vi "Test write read.vi"() -> ()   [LabVIEW 2021]
uses:
  TypeDefs/Read Configuration.ctl
  TypeDefs/Read Position.ctl
  TypeDefs/Data Element Details.ctl
  2e8eb7a4-6c45-41fc-8a56-8b93f8ab2aed.vi
  1e1cc0e0-5587-4368-b9c8-22ab8a2609bf.vi
  124ed0cf-21a2-4029-8b72-d8b2bc3cfca2.vi
  5f672ce3-c1c3-4239-be86-591df5452e6b.vi
  7cfac513-7288-4c82-908e-0b73a446185f.vi
  0aeae9fb-4646-413c-b569-2ea3bfc416eb.vi
  83090dc5-7c38-4dd0-9690-bbdffacb842e.vi
  30ab5228-805b-4106-80f0-7bddeadb9d94.vi
  0f7b4db4-c933-4198-9d44-a71b046c91fc.vi
  fd82cae6-90a1-4db4-8629-0dfa001c7628.vi
  3a8d97a0-d580-4512-a7c4-2f0697e6c9e2.vi
  132e0870-f3bc-4a70-93a8-8291f934a74e.vi
  1a26c85e-4bdf-40ac-9bb8-9f3aeb47762f.vi
  fc566840-9c7d-4747-891b-faea8883fc20.vi
  4087863d-db22-4010-a15b-9626b6b88f25.vi
  5d30ffee-c7bc-441f-904d-ba5baae4ab9b.vi
  5997d33c-b1c7-4e50-8cd9-5e7827217409.vi
  1b0a551c-ab50-4056-a338-be00ced168a1.vi
  1475facd-0be5-4a16-b5c0-d4b4098ff17d.vi
  2d2b7dd1-084a-416f-9403-29da1a0cacdf.vi
  71538749-b1ea-46d3-91f5-b8a08187b131.vi
  7ca0a5c6-c913-495e-bc60-1e54ff021bc4.vi
  0c9d9d69-203a-4c45-ab83-8723ccfac58a.vi
  8b09acb3-1804-4adb-b57a-6ab97de36fae.vi
  41820140-f02b-403e-8f6d-e5d8cc9e6038.vi
  5fe378b5-e28f-447f-911b-385a06e12749.vi
  6975467f-3c1c-408b-9985-6bf92f704002.vi
  a5ee0e2d-1d32-4a5c-9f8c-ab7e37a9bb32.vi
  6e041348-7f94-4adb-a506-9e6ae80f31c7.vi
  287dc7c8-fd1f-4848-acac-6b048d61fa92.vi
  96fd03da-6166-4d98-b503-d6d912d62be1.vi
  cd5f71e7-aa80-496b-a46f-ff9cfb96c09e.vi
  ab81dfaa-b4ed-4dad-90db-c2069a499ab9.vi
  cdd1d806-cf03-48b9-80a7-5abb69cc969c.vi
  934c8ee6-8108-47c3-ab0c-e7f3872857de.vi
  0617b4dd-75f0-4fc1-be0a-72d777f45d9a.vi
  6dbf1ba6-5076-4e89-aafa-fa0408d53c9c.vi
  87883e52-c370-4e1d-99dd-8208e79277b9.vi
  5a5884df-cfb3-4237-a45a-462ccf1dc42e.vi
  d4ea617a-d912-406f-a3a4-9dbd6f53576b.vi
  305478fb-600b-4089-8c06-0e062707fa97.vi
  44847041-c2b7-4435-a919-9d7ef56b5811.vi
  442734bb-6a94-4929-a174-6a0af52723c3.vi
  37e1ea89-1b34-4e4e-9bfd-fc0f3fde4930.vi
  2b752281-b4de-4725-8373-b94f73551aa8.vi
  2e8eb7a4-6c45-41fc-8a56-8b93f8ab2aed.vi/49b3dd2d-4579-4089-b72e-3f0875c862f2.vi
  SubVIs/Check Error.vi
  SubVIs/Get dll Path.vi
  SubVIs/Get Element Write Position.vi
  SubVIs/Notify Of New Write.vi
  124ed0cf-21a2-4029-8b72-d8b2bc3cfca2.vi/ad4ed45e-f2aa-403d-a38b-be52afbcecdf.vi
  5f672ce3-c1c3-4239-be86-591df5452e6b.vi/49b3dd2d-4579-4089-b72e-3f0875c862f2.vi
  0aeae9fb-4646-413c-b569-2ea3bfc416eb.vi/ad4ed45e-f2aa-403d-a38b-be52afbcecdf.vi
  83090dc5-7c38-4dd0-9690-bbdffacb842e.vi/bd07d5d9-1209-45ad-b636-9e9ab86132fb.vi
  0f7b4db4-c933-4198-9d44-a71b046c91fc.vi/ad4ed45e-f2aa-403d-a38b-be52afbcecdf.vi
  fd82cae6-90a1-4db4-8629-0dfa001c7628.vi/bd07d5d9-1209-45ad-b636-9e9ab86132fb.vi
  132e0870-f3bc-4a70-93a8-8291f934a74e.vi/ad4ed45e-f2aa-403d-a38b-be52afbcecdf.vi
  1a26c85e-4bdf-40ac-9bb8-9f3aeb47762f.vi/49b3dd2d-4579-4089-b72e-3f0875c862f2.vi
  4087863d-db22-4010-a15b-9626b6b88f25.vi/ad4ed45e-f2aa-403d-a38b-be52afbcecdf.vi
  5d30ffee-c7bc-441f-904d-ba5baae4ab9b.vi/ad4ed45e-f2aa-403d-a38b-be52afbcecdf.vi
  5997d33c-b1c7-4e50-8cd9-5e7827217409.vi/49b3dd2d-4579-4089-b72e-3f0875c862f2.vi
  2d2b7dd1-084a-416f-9403-29da1a0cacdf.vi/ad4ed45e-f2aa-403d-a38b-be52afbcecdf.vi
  71538749-b1ea-46d3-91f5-b8a08187b131.vi/ad4ed45e-f2aa-403d-a38b-be52afbcecdf.vi
  7ca0a5c6-c913-495e-bc60-1e54ff021bc4.vi/49b3dd2d-4579-4089-b72e-3f0875c862f2.vi
  41820140-f02b-403e-8f6d-e5d8cc9e6038.vi/ad4ed45e-f2aa-403d-a38b-be52afbcecdf.vi
  5fe378b5-e28f-447f-911b-385a06e12749.vi/ad4ed45e-f2aa-403d-a38b-be52afbcecdf.vi
  6975467f-3c1c-408b-9985-6bf92f704002.vi/49b3dd2d-4579-4089-b72e-3f0875c862f2.vi
  6e041348-7f94-4adb-a506-9e6ae80f31c7.vi/ad4ed45e-f2aa-403d-a38b-be52afbcecdf.vi
  287dc7c8-fd1f-4848-acac-6b048d61fa92.vi/ad4ed45e-f2aa-403d-a38b-be52afbcecdf.vi
  96fd03da-6166-4d98-b503-d6d912d62be1.vi/49b3dd2d-4579-4089-b72e-3f0875c862f2.vi
  ab81dfaa-b4ed-4dad-90db-c2069a499ab9.vi/ad4ed45e-f2aa-403d-a38b-be52afbcecdf.vi
  cdd1d806-cf03-48b9-80a7-5abb69cc969c.vi/49b3dd2d-4579-4089-b72e-3f0875c862f2.vi
  0617b4dd-75f0-4fc1-be0a-72d777f45d9a.vi/ad4ed45e-f2aa-403d-a38b-be52afbcecdf.vi
  6dbf1ba6-5076-4e89-aafa-fa0408d53c9c.vi/49b3dd2d-4579-4089-b72e-3f0875c862f2.vi
  87883e52-c370-4e1d-99dd-8208e79277b9.vi/49b3dd2d-4579-4089-b72e-3f0875c862f2.vi
  5a5884df-cfb3-4237-a45a-462ccf1dc42e.vi/49b3dd2d-4579-4089-b72e-3f0875c862f2.vi
  SubVIs/Wait For N Elements Available.vi
  SubVIs/Get Element Read Position.vi
  SubVIs/Set Element Read Position.vi
  442734bb-6a94-4929-a174-6a0af52723c3.vi/49b3dd2d-4579-4089-b72e-3f0875c862f2.vi
  2b752281-b4de-4725-8373-b94f73551aa8.vi/ad4ed45e-f2aa-403d-a38b-be52afbcecdf.vi
  <vilib>/Utility/error.llb/Trim Whitespace.vi
  <vilib>/string/Create NI GUID.vi
  <vilib>/Utility/error.llb/Error Cluster From Error Code.vi
  SubVIs/Get Element Info Variant.vi
  CIF_NI_CIPC.lvlib
panel:
  out "status":string
  out "pass":bool
  out "error out":errorcluster
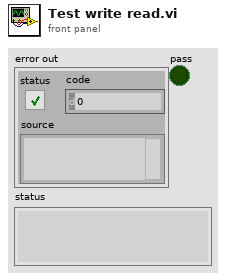
[diagram p1: front panel]
types:
  T1 = typedef "CIF_NI_CIPC.lvlib/Data Element Details.ctl" = cluster{"Bytes to Read":u32, "Element Offset":u32}
  T2 = cluster{"U16":u16, "I32":i32, bool, "embedded":cluster{dbl, "bool":bool}}
  T3 = typedef "Read Result Details.ctl" = cluster{"Array Size":i32, "Element Offset Last Read":u32, "Overwritten":bool}
  T4 = typedef "Read Configuration.ctl" = cluster{"Read Position (Newest)":T5, "Element Offset":i32, "Prepend Array Size":bool, "Get Read Position":bool}
  T5 = typedef "CIF_NI_CIPC.lvlib/Read Position.ctl" = enum16{"Next", "Newest", "Oldest", "Next Available", "Absolute"}
  T6 = typedef "CIF_NI_CIPC.lvlib/Encoder Info.ctl" = cluster{"Name":string, "Version":i32, "Data":string}
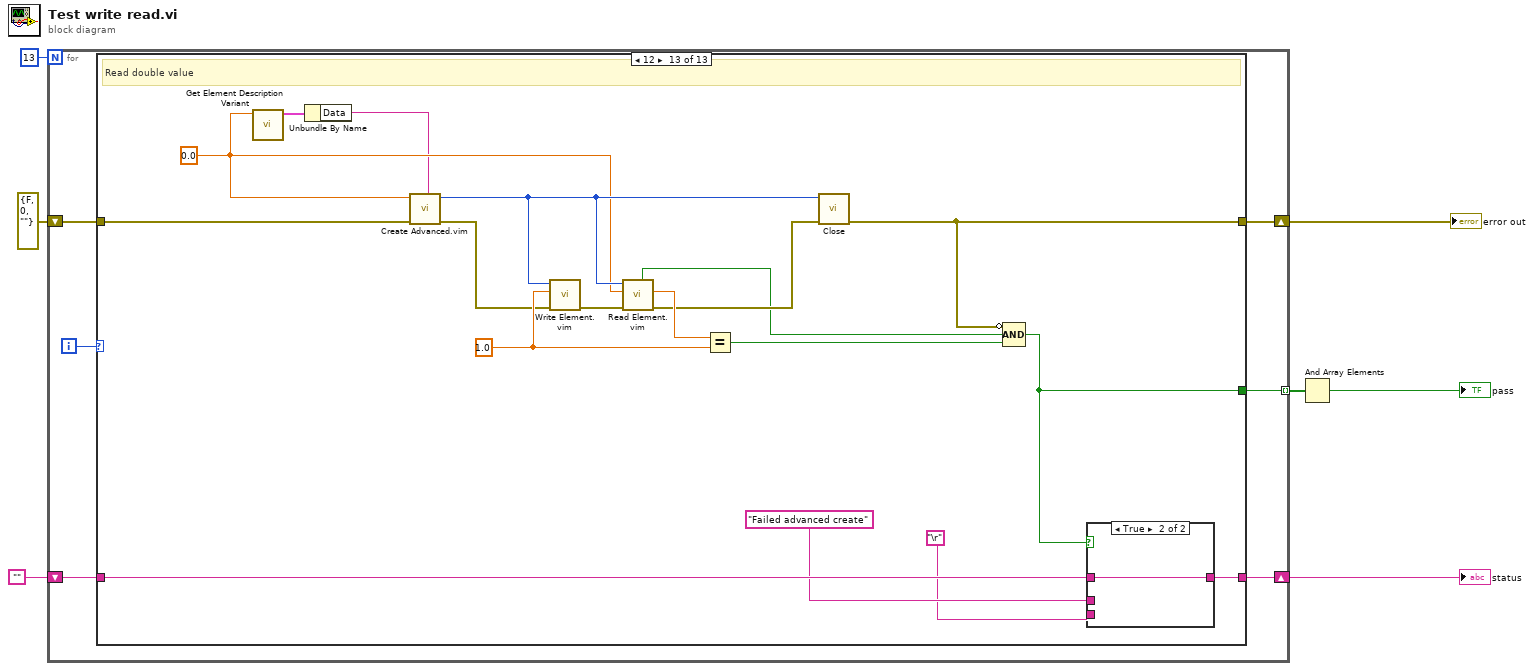
[diagram p0: block diagram]
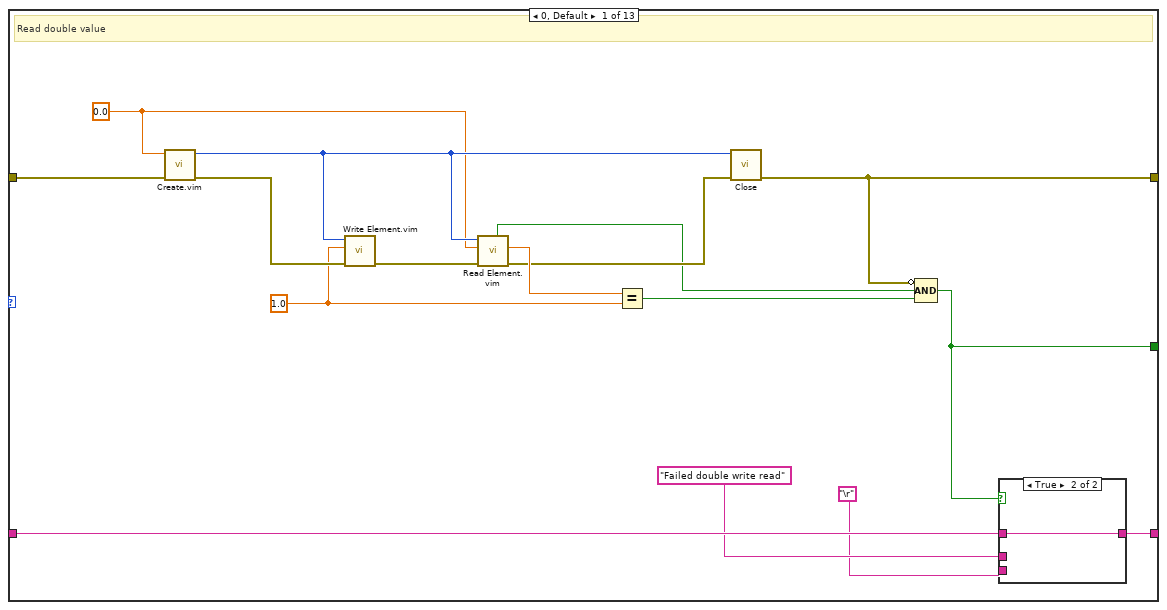
[diagram p2: hidden frame]
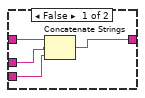
[diagram p3: hidden frame]
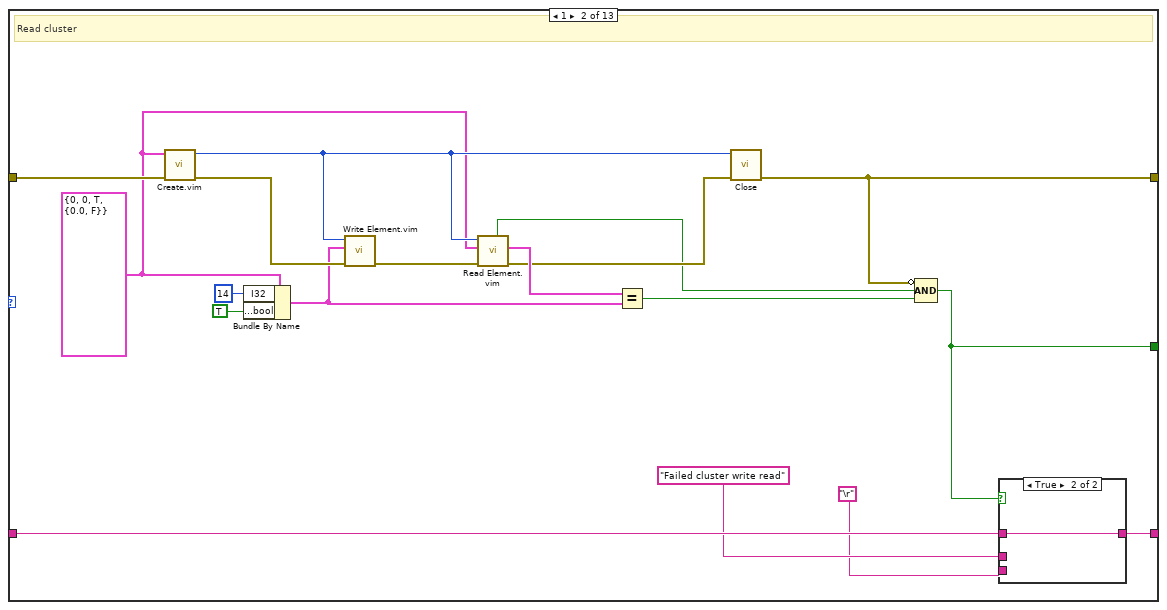
[diagram p4: hidden frame]
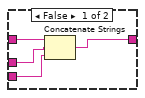
[diagram p5: hidden frame]
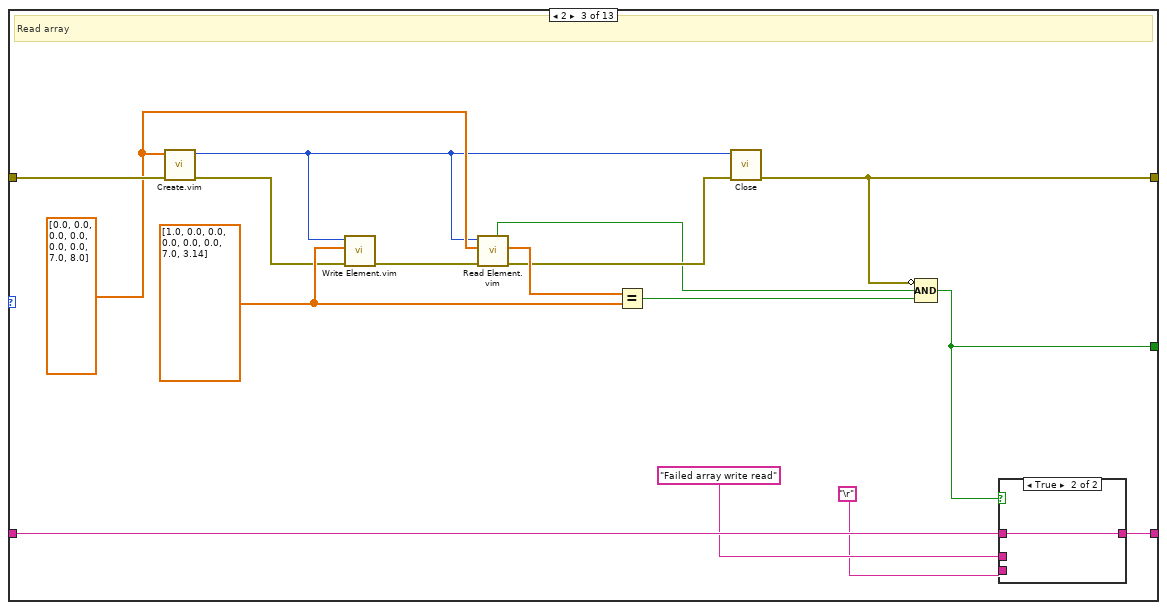
[diagram p6: hidden frame]
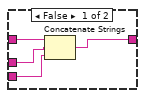
[diagram p7: hidden frame]
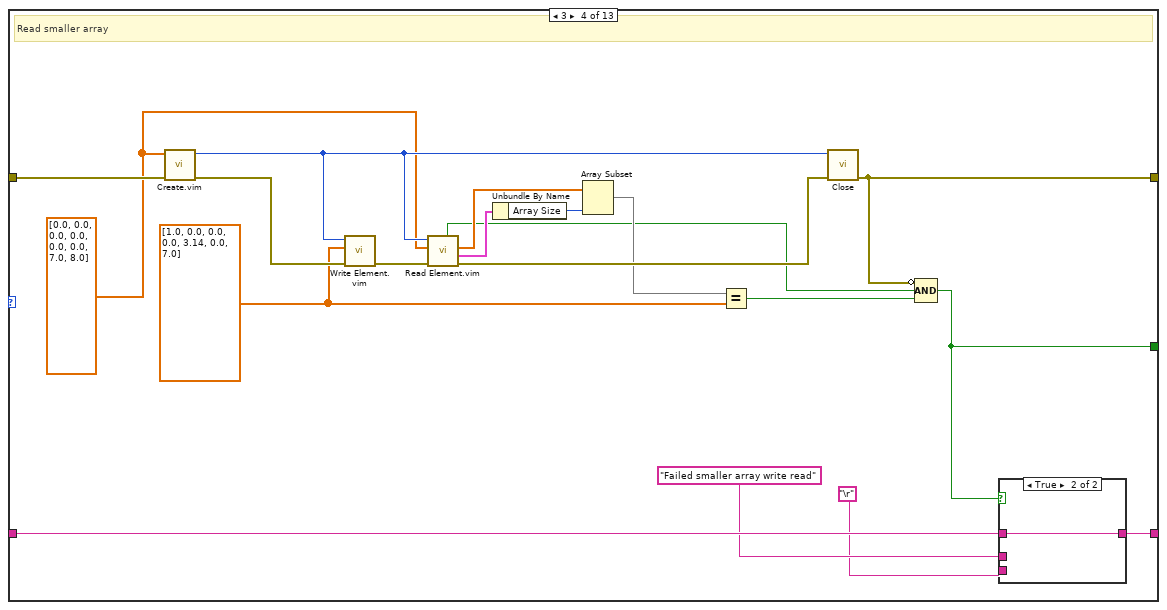
[diagram p8: hidden frame]
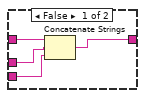
[diagram p9: hidden frame]
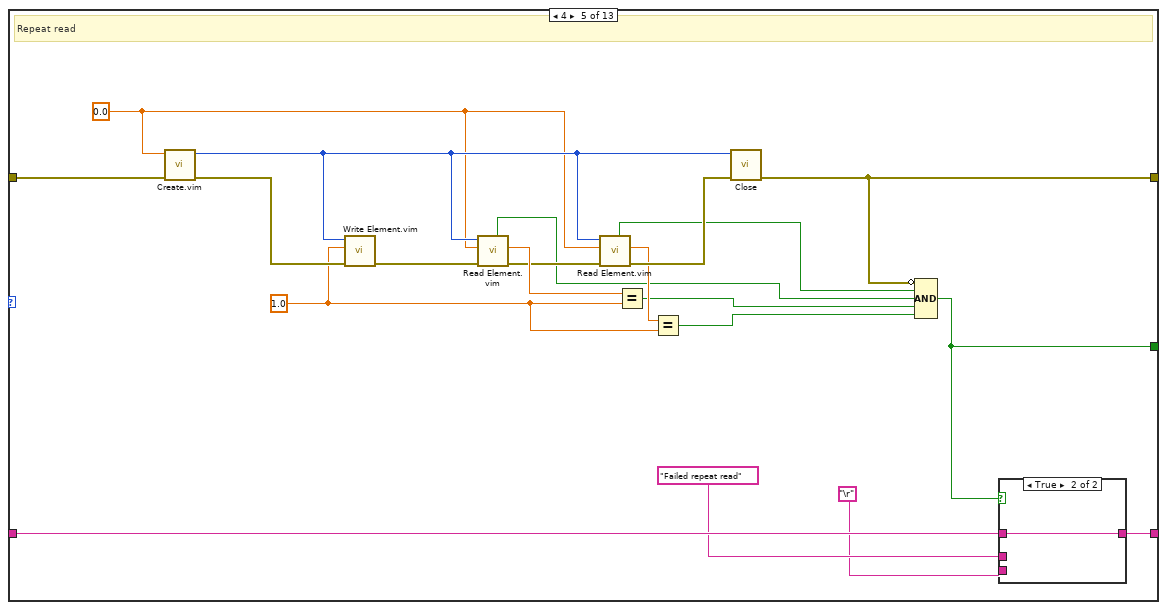
[diagram p10: hidden frame]
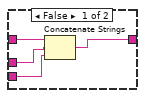
[diagram p11: hidden frame]
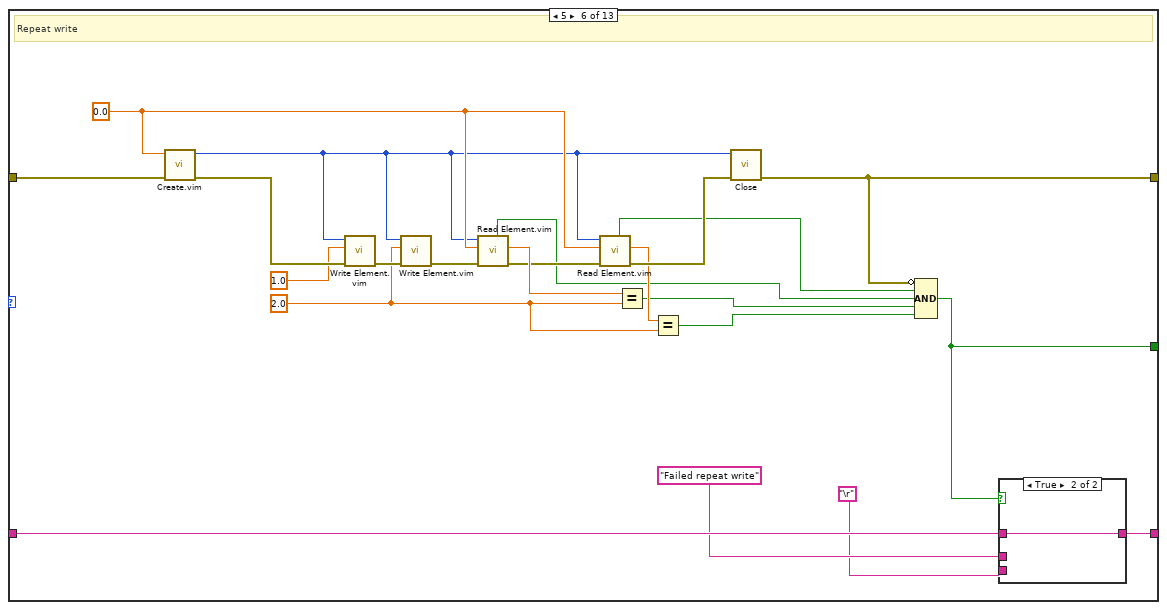
[diagram p12: hidden frame]
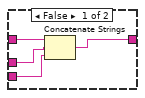
[diagram p13: hidden frame]
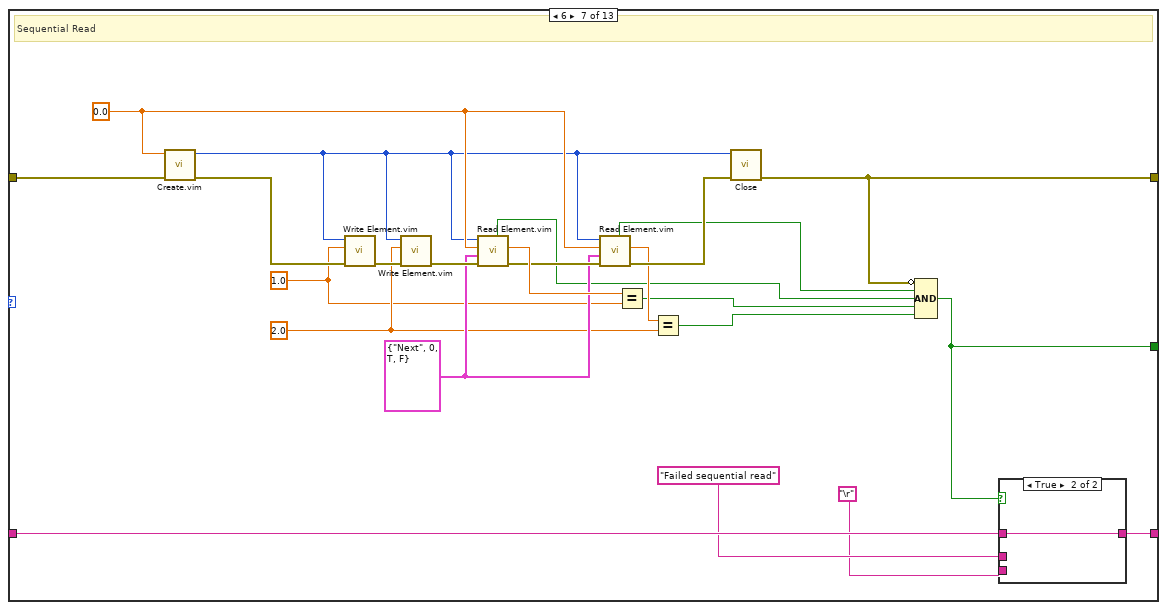
[diagram p14: hidden frame]
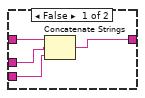
[diagram p15: hidden frame]
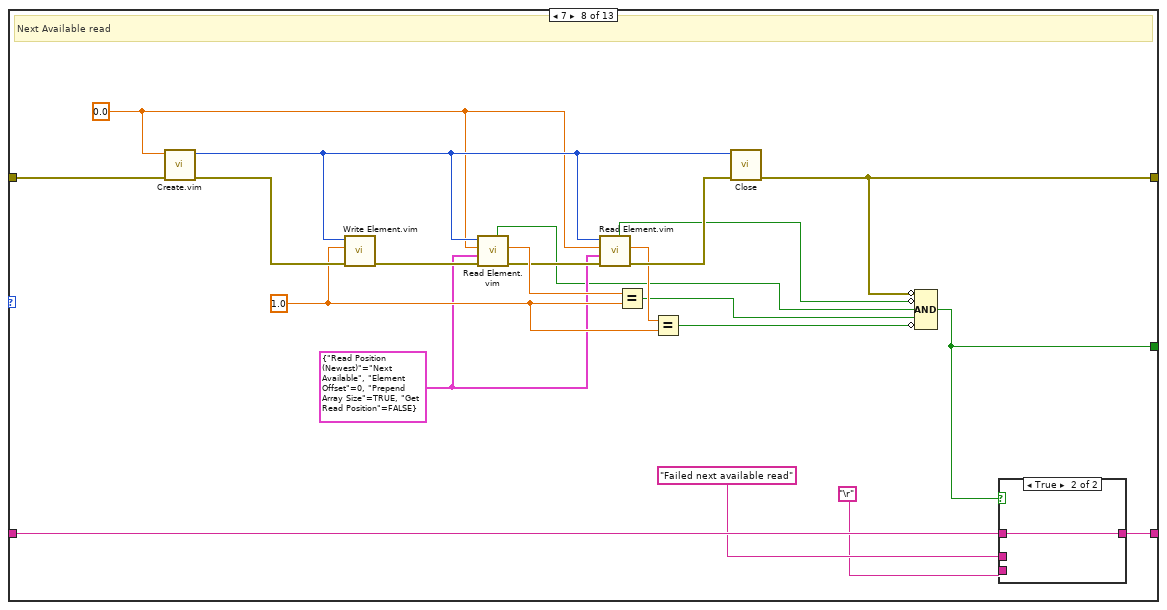
[diagram p16: hidden frame]
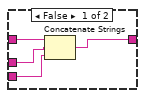
[diagram p17: hidden frame]
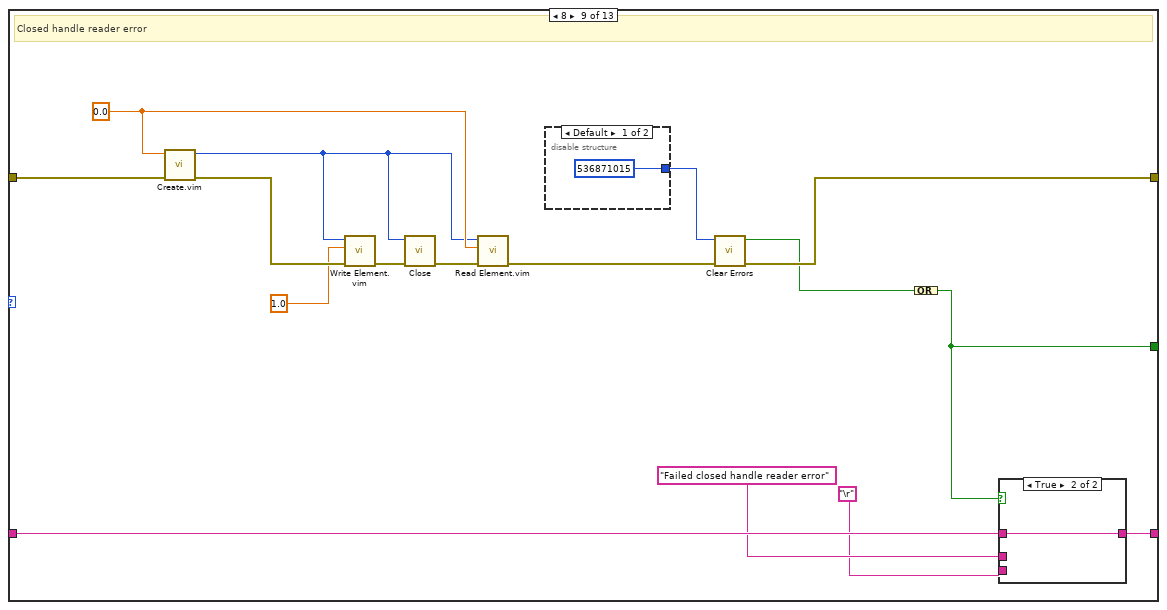
[diagram p18: hidden frame]
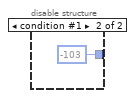
[diagram p19: hidden frame]
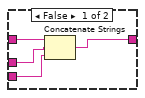
[diagram p20: hidden frame]
diagram:
  n1 = for {
    N: 13 -> [_]
    tunnel: [w13] -> w7 mode=indexing
    shift-right: [w10] -> w3
    shift-left: "" -> [w11]
    shift-right: [w9] -> w1
    shift-left: errorcluster {"status"=FALSE, "code"=0, "source"=""} ("error out") -> [w8]
    i -> [w12]
    n2 = case shown="12" w12 {
      tunnel: [w25 w48 w69 w93 w118 w145 w173 w199 w220 w243 w265 w297 w320] -> w13
      tunnel: w11 -> [w29 w52 w73 w97 w122 w149 w177 w203 w224 w247 w269 w301 w324]
      tunnel: [w28 w51 w72 w96 w121 w148 w176 w202 w223 w246 w268 w300 w323] -> w10
      tunnel: [w16 w41 w64 w87 w114 w142 w170 w195 w212 w238 w255 w284 w314] -> w9
      tunnel: w8 -> [w15 w40 w63 w86 w113 w141 w169 w194 w216 w240 w263 w285 w312]
      frame 0, Default {
        w19 = 1.0
        w18 = 0.0
        # "Read double value"
        n3 = call "Create.vim"("error in (no error)"=w15, "Data Type"=w18) -> ("error out"=w24:errorcluster, "CIPC Reference"=w23:u64)  [unwired: 6 in, 2 out]
        n4 = call "Write Element.vim"("error in (no error)"=w24, "Data in"=w19, "CIPC Reference in"=w23) -> ("error out"=w22:errorcluster)  [unwired: 5 in, 3 out]
        n5 = call "Read Element.vim"("error in"=w22, "Data in"=w18, "CIPC Reference in"=w23) -> ("error out"=w20:errorcluster, "Data out"=w21:dbl, "Success"=w14:bool)  [unwired: 4 in, 2 out]
        n6 = Equal?(x=w21, y=w19) -> (x = y?=w17:bool)
        n7 = call "Close.vi"("error in (no error)"=w20, "CIPC Reference"=w23) -> ("error out"=w16:errorcluster)  [unwired: 9 in]
        n8 = Compound Arithmetic op=AND(invert w16, w14, w17) -> (w25:bool)
        n9 = case shown="True" w25 {
          tunnel: w29 -> [w33 w34]
          tunnel: [w30 w34] -> w28
          tunnel: "Failed double write read" -> [w32 _]
          tunnel: "\r" -> [w31 _]
          frame False {
            n10 = Concatenate Strings(w33, w32, w31) -> (w30:string)
          }
          frame True {
          }
        }
      }
      frame 1 {
        w39 = T2 {"U16"=0, "I32"=0, TRUE, "embedded"={0.0, "bool"=FALSE}}
        # "Read cluster"
        n11 = call "Create.vim"("error in (no error)"=w40, "Data Type"=w39) -> ("error out"=w47:errorcluster, "CIPC Reference"=w46:u64)  [unwired: 6 in, 2 out]
        n12 = Bundle By Name(cluster=w39, "I32"=14, "embedded.bool"=TRUE) -> (w38:T2)
        n13 = call "Write Element.vim"("error in (no error)"=w47, "Data in"=w38, "CIPC Reference in"=w46) -> ("error out"=w45:errorcluster)  [unwired: 5 in, 3 out]
        n14 = call "Read Element.vim"("error in"=w45, "Data in"=w39, "CIPC Reference in"=w46) -> ("error out"=w43:errorcluster, "Data out"=w44:T2, "Success"=w35:bool)  [unwired: 4 in, 2 out]
        n15 = Equal?(x=w44, y=w38) -> (x = y?=w42:bool)
        n16 = call "Close.vi"("error in (no error)"=w43, "CIPC Reference"=w46) -> ("error out"=w41:errorcluster)  [unwired: 9 in]
        n17 = Compound Arithmetic op=AND(invert w41, w35, w42) -> (w48:bool)
        n18 = case shown="True" w48 {
          tunnel: w52 -> [w56 w57]
          tunnel: [w53 w57] -> w51
          tunnel: "Failed cluster write read" -> [w55 _]
          tunnel: "\r" -> [w54 _]
          frame False {
            n19 = Concatenate Strings(w56, w55, w54) -> (w53:string)
          }
          frame True {
          }
        }
      }
      frame 2 {
        w61 = dbl[] [1.0, 0.0, 0.0, 0.0, 0.0, 0.0, 7.0, 3.14]
        w62 = dbl[] [0.0, 0.0, 0.0, 0.0, 0.0, 0.0, 7.0, 8.0]
        # "Read array"
        n20 = call "Create.vim"("error in (no error)"=w63, "Data Type"=w62) -> ("error out"=w60:errorcluster, "CIPC Reference"=w59:u64)  [unwired: 6 in, 2 out]
        n21 = call "Write Element.vim"("error in (no error)"=w60, "Data in"=w61, "CIPC Reference in"=w59) -> ("error out"=w68:errorcluster)  [unwired: 5 in, 3 out]
        n22 = call "Read Element.vim"("error in"=w68, "Data in"=w62, "CIPC Reference in"=w59) -> ("error out"=w66:errorcluster, "Data out"=w67:dbl[], "Success"=w58:bool)  [unwired: 4 in, 2 out]
        n23 = Equal?(x=w67, y=w61) -> (x = y?=w65:bool)
        n24 = call "Close.vi"("error in (no error)"=w66, "CIPC Reference"=w59) -> ("error out"=w64:errorcluster)  [unwired: 9 in]
        n25 = Compound Arithmetic op=AND(invert w64, w58, w65) -> (w69:bool)
        n26 = case shown="True" w69 {
          tunnel: w73 -> [w77 w78]
          tunnel: [w74 w78] -> w72
          tunnel: "Failed array write read" -> [w76 _]
          tunnel: "\r" -> [w75 _]
          frame False {
            n27 = Concatenate Strings(w77, w76, w75) -> (w74:string)
          }
          frame True {
          }
        }
      }
      frame 3 {
        w84 = dbl[] [1.0, 0.0, 0.0, 0.0, 3.14, 0.0, 7.0]
        w85 = dbl[] [0.0, 0.0, 0.0, 0.0, 0.0, 0.0, 7.0, 8.0]
        # "Read smaller array"
        n28 = call "Create.vim"("error in (no error)"=w86, "Data Type"=w85) -> ("error out"=w92:errorcluster, "CIPC Reference"=w91:u64)  [unwired: 6 in, 2 out]
        n29 = call "Write Element.vim"("error in (no error)"=w92, "Data in"=w84, "CIPC Reference in"=w91) -> ("error out"=w90:errorcluster)  [unwired: 5 in, 3 out]
        n30 = call "Read Element.vim"("error in"=w90, "Data in"=w85, "CIPC Reference in"=w91) -> ("error out"=w89:errorcluster, "Read Result Details"=w83:T3, "Data out"=w82:dbl[], "Success"=w79:bool)  [unwired: 4 in, 1 out]
        n31 = Unbundle By Name(w83) -> ("Array Size"=w81:i32)
        n32 = Array Subset(array=w82, length=w81) -> (w80:dbl[])  [unwired: 1 in]
        n33 = Equal?(x=w80, y=w84) -> (x = y?=w88:bool)
        n34 = call "Close.vi"("error in (no error)"=w89, "CIPC Reference"=w91) -> ("error out"=w87:errorcluster)  [unwired: 9 in]
        n35 = Compound Arithmetic op=AND(invert w87, w79, w88) -> (w93:bool)
        n36 = case shown="True" w93 {
          tunnel: w97 -> [w101 w102]
          tunnel: [w98 w102] -> w96
          tunnel: "Failed smaller array write read" -> [w100 _]
          tunnel: "\r" -> [w99 _]
          frame False {
            n37 = Concatenate Strings(w101, w100, w99) -> (w98:string)
          }
          frame True {
          }
        }
      }
      frame 4 {
        w107 = 1.0
        w108 = 0.0
        # "Repeat read"
        n38 = call "Create.vim"("error in (no error)"=w113, "Data Type"=w108) -> ("error out"=w117:errorcluster, "CIPC Reference"=w112:u64)  [unwired: 6 in, 2 out]
        n39 = call "Write Element.vim"("error in (no error)"=w117, "Data in"=w107, "CIPC Reference in"=w112) -> ("error out"=w116:errorcluster)  [unwired: 5 in, 3 out]
        n40 = call "Read Element.vim"("error in"=w116, "Data in"=w108, "CIPC Reference in"=w112) -> ("error out"=w111:errorcluster, "Data out"=w115:dbl, "Success"=w104:bool)  [unwired: 4 in, 2 out]
        n41 = call "Read Element.vim"("error in"=w111, "Data in"=w108, "CIPC Reference in"=w112) -> ("error out"=w110:errorcluster, "Data out"=w109:dbl, "Success"=w103:bool)  [unwired: 4 in, 2 out]
        n42 = Equal?(x=w115, y=w107) -> (x = y?=w105:bool)
        n43 = Equal?(x=w109, y=w107) -> (x = y?=w106:bool)
        n44 = call "Close.vi"("error in (no error)"=w110, "CIPC Reference"=w112) -> ("error out"=w114:errorcluster)  [unwired: 9 in]
        n45 = Compound Arithmetic op=AND(invert w114, w103, w104, w105, w106) -> (w118:bool)
        n46 = case shown="True" w118 {
          tunnel: w122 -> [w126 w127]
          tunnel: [w123 w127] -> w121
          tunnel: "Failed repeat read" -> [w125 _]
          tunnel: "\r" -> [w124 _]
          frame False {
            n47 = Concatenate Strings(w126, w125, w124) -> (w123:string)
          }
          frame True {
          }
        }
      }
      frame 5 {
        w130 = 2.0
        w137 = 0.0
        # "Repeat write"
        n48 = call "Create.vim"("error in (no error)"=w141, "Data Type"=w137) -> ("error out"=w144:errorcluster, "CIPC Reference"=w132:u64)  [unwired: 6 in, 2 out]
        n49 = call "Write Element.vim"("error in (no error)"=w144, "Data in"=1.0, "CIPC Reference in"=w132) -> ("error out"=w134:errorcluster)  [unwired: 5 in, 3 out]
        n50 = call "Write Element.vim"("error in (no error)"=w134, "Data in"=w130, "CIPC Reference in"=w132) -> ("error out"=w133:errorcluster)  [unwired: 5 in, 3 out]
        n51 = call "Read Element.vim"("error in"=w133, "Data in"=w137, "CIPC Reference in"=w132) -> ("error out"=w140:errorcluster, "Data out"=w143:dbl, "Success"=w129:bool)  [unwired: 4 in, 2 out]
        n52 = call "Read Element.vim"("error in"=w140, "Data in"=w137, "CIPC Reference in"=w132) -> ("error out"=w139:errorcluster, "Data out"=w138:dbl, "Success"=w128:bool)  [unwired: 4 in, 2 out]
        n53 = Equal?(x=w143, y=w130) -> (x = y?=w135:bool)
        n54 = Equal?(x=w138, y=w130) -> (x = y?=w136:bool)
        n55 = call "Close.vi"("error in (no error)"=w139, "CIPC Reference"=w132) -> ("error out"=w142:errorcluster)  [unwired: 9 in]
        n56 = Compound Arithmetic op=AND(invert w142, w128, w129, w135, w136) -> (w145:bool)
        n57 = case shown="True" w145 {
          tunnel: w149 -> [w153 w154]
          tunnel: [w150 w154] -> w148
          tunnel: "Failed repeat write" -> [w152 _]
          tunnel: "\r" -> [w151 _]
          frame False {
            n58 = Concatenate Strings(w153, w152, w151) -> (w150:string)
          }
          frame True {
          }
        }
      }
      frame 6 {
        w159 = T4 {"Read Position (Newest)"=enum."Next", "Element Offset"=0, "Prepend Array Size"=TRUE, "Get Read Position"=FALSE} ("Read Configuration")
        w157 = 1.0
        w158 = 2.0
        w165 = 0.0
        # "Sequential Read"
        n59 = call "Create.vim"("error in (no error)"=w169, "Data Type"=w165) -> ("error out"=w172:errorcluster, "CIPC Reference"=w160:u64)  [unwired: 6 in, 2 out]
        n60 = call "Write Element.vim"("error in (no error)"=w172, "Data in"=w157, "CIPC Reference in"=w160) -> ("error out"=w162:errorcluster)  [unwired: 5 in, 3 out]
        n61 = call "Write Element.vim"("error in (no error)"=w162, "Data in"=w158, "CIPC Reference in"=w160) -> ("error out"=w161:errorcluster)  [unwired: 5 in, 3 out]
        n62 = call "Read Element.vim"("error in"=w161, "Read Configuration"=w159, "Data in"=w165, "CIPC Reference in"=w160) -> ("error out"=w168:errorcluster, "Data out"=w171:dbl, "Success"=w156:bool)  [unwired: 3 in, 2 out]
        n63 = call "Read Element.vim"("error in"=w168, "Read Configuration"=w159, "Data in"=w165, "CIPC Reference in"=w160) -> ("error out"=w167:errorcluster, "Data out"=w166:dbl, "Success"=w155:bool)  [unwired: 3 in, 2 out]
        n64 = Equal?(x=w171, y=w157) -> (x = y?=w163:bool)
        n65 = Equal?(x=w166, y=w158) -> (x = y?=w164:bool)
        n66 = call "Close.vi"("error in (no error)"=w167, "CIPC Reference"=w160) -> ("error out"=w170:errorcluster)  [unwired: 9 in]
        n67 = Compound Arithmetic op=AND(invert w170, w155, w156, w163, w164) -> (w173:bool)
        n68 = case shown="True" w173 {
          tunnel: w177 -> [w181 w182]
          tunnel: [w178 w182] -> w176
          tunnel: "Failed sequential read" -> [w180 _]
          tunnel: "\r" -> [w179 _]
          frame False {
            n69 = Concatenate Strings(w181, w180, w179) -> (w178:string)
          }
          frame True {
          }
        }
      }
      frame 7 {
        w185 = T4 {"Read Position (Newest)"=enum."Next Available", "Element Offset"=0, "Prepend Array Size"=TRUE, "Get Read Position"=FALSE} ("Read Configuration")
        w188 = 1.0
        w189 = 0.0
        # "Next Available read"
        n70 = call "Create.vim"("error in (no error)"=w194, "Data Type"=w189) -> ("error out"=w198:errorcluster, "CIPC Reference"=w193:u64)  [unwired: 6 in, 2 out]
        n71 = call "Write Element.vim"("error in (no error)"=w198, "Data in"=w188, "CIPC Reference in"=w193) -> ("error out"=w197:errorcluster)  [unwired: 5 in, 3 out]
        n72 = call "Read Element.vim"("error in"=w197, "Read Configuration"=w185, "Data in"=w189, "CIPC Reference in"=w193) -> ("error out"=w192:errorcluster, "Data out"=w196:dbl, "Success"=w184:bool)  [unwired: 3 in, 2 out]
        n73 = call "Read Element.vim"("error in"=w192, "Read Configuration"=w185, "Data in"=w189, "CIPC Reference in"=w193) -> ("error out"=w191:errorcluster, "Data out"=w190:dbl, "Success"=w183:bool)  [unwired: 3 in, 2 out]
        n74 = Equal?(x=w196, y=w188) -> (x = y?=w186:bool)
        n75 = Equal?(x=w190, y=w188) -> (x = y?=w187:bool)
        n76 = call "Close.vi"("error in (no error)"=w191, "CIPC Reference"=w193) -> ("error out"=w195:errorcluster)  [unwired: 9 in]
        n77 = Compound Arithmetic op=AND(invert w195, invert w183, w184, w186, invert w187) -> (w199:bool)
        n78 = case shown="True" w199 {
          tunnel: w203 -> [w207 w208]
          tunnel: [w204 w208] -> w202
          tunnel: "Failed next available read" -> [w206 _]
          tunnel: "\r" -> [w205 _]
          frame False {
            n79 = Concatenate Strings(w207, w206, w205) -> (w204:string)
          }
          frame True {
          }
        }
      }
      frame 8 {
        w217 = 0.0
        # "Closed handle reader error"
        n80 = call "Create.vim"("error in (no error)"=w216, "Data Type"=w217) -> ("error out"=w219:errorcluster, "CIPC Reference"=w213:u64)  [unwired: 6 in, 2 out]
        n81 = call "Write Element.vim"("error in (no error)"=w219, "Data in"=1.0, "CIPC Reference in"=w213) -> ("error out"=w215:errorcluster)  [unwired: 5 in, 3 out]
        n82 = call "Close.vi"("error in (no error)"=w215, "CIPC Reference"=w213) -> ("error out"=w214:errorcluster)  [unwired: 9 in]
        n83 = call "Read Element.vim"("error in"=w214, "Data in"=w217, "CIPC Reference in"=w213) -> ("error out"=w209:errorcluster)  [unwired: 4 in, 4 out]
        n84 = disable-structure shown="Default" {
          disable-tunnel: [536871015 ("specific error code to clear (0: all)") -103 ("specific error code to clear (0: all)")] -> w211
          frame condition #0 (active) {
          }
          frame condition #1 {
          }
        }
        n85 = call <vilib>:"Clear Errors.vi"("error in (no error)"=w209, "specific error code to clear (0: all)"=w211) -> ("error out"=w212:errorcluster, "specific error cleared?"=w210:bool)  [unwired: 4 in]
        n86 = Compound Arithmetic op=OR(w210) -> (w220:bool)
        n87 = case shown="True" w220 {
          tunnel: w224 -> [w230 w231]
          tunnel: [w227 w231] -> w223
          tunnel: "Failed closed handle reader error" -> [w229 _]
          tunnel: "\r" -> [w228 _]
          frame False {
            n88 = Concatenate Strings(w230, w229, w228) -> (w227:string)
          }
          frame True {
          }
        }
      }
      frame 9 {
        w241 = 0.0
        # "Closed handle error writer"
        n89 = call "Create.vim"("error in (no error)"=w240, "Data Type"=w241) -> ("error out"=w234:errorcluster, "CIPC Reference"=w235:u64)  [unwired: 6 in, 2 out]
        n90 = call "Close.vi"("error in (no error)"=w234, "CIPC Reference"=w235) -> ("error out"=w233:errorcluster)  [unwired: 9 in]
        n91 = call "Write Element.vim"("error in (no error)"=w233, "Data in"=1.0, "CIPC Reference in"=w235) -> ("error out"=w232:errorcluster)  [unwired: 5 in, 3 out]
        n92 = call "Read Element.vim"("error in"=w232, "Data in"=w241, "CIPC Reference in"=w235) -> ("error out"=w239:errorcluster)  [unwired: 4 in, 4 out]
        n93 = disable-structure shown="TARGET_TYPE==RT" {
          disable-tunnel: [536871015 ("specific error code to clear (0: all)") -103 ("specific error code to clear (0: all)")] -> w237
          frame condition #0 (active) {
          }
          frame condition #1 {
          }
        }
        n94 = call <vilib>:"Clear Errors.vi"("error in (no error)"=w239, "specific error code to clear (0: all)"=w237) -> ("error out"=w238:errorcluster, "specific error cleared?"=w236:bool)  [unwired: 4 in]
        n95 = Compound Arithmetic op=AND(w236) -> (w243:bool)
        n96 = case shown="True" w243 {
          tunnel: w247 -> [w253 w254]
          tunnel: [w250 w254] -> w246
          tunnel: "Failed closed handle writer error" -> [w252 _]
          tunnel: "\r" -> [w251 _]
          frame False {
            n97 = Concatenate Strings(w253, w252, w251) -> (w250:string)
          }
          frame True {
          }
        }
      }
      frame 10 {
        w259 = "testme" ("Name in")
        # "Closed and reuse name"
        n98 = call "Create.vim"("error in (no error)"=w263, "Name in"=w259, "Data Type"=0.0) -> ("error out"=w257:errorcluster, "CIPC Reference"=w258:u64)  [unwired: 5 in, 2 out]
        n99 = call "Close.vi"("error in (no error)"=w257, "CIPC Reference"=w258) -> ("error out"=w256:errorcluster)  [unwired: 9 in]
        n100 = call "Create.vim"("error in (no error)"=w256, "Name in"=w259, "Data Type"=0) -> ("error out"=w261:errorcluster, "CIPC Reference"=w260:u64)  [unwired: 5 in, 2 out]
        n101 = call "Close.vi"("error in (no error)"=w261, "CIPC Reference"=w260) -> ("error out"=w255:errorcluster)  [unwired: 9 in]
        n102 = Compound Arithmetic op=AND(invert w255) -> (w265:bool)
        n103 = case shown="True" w265 {
          tunnel: w269 -> [w273 w274]
          tunnel: [w270 w274] -> w268
          tunnel: "Failed reuse name" -> [w272 _]
          tunnel: "\r" -> [w271 _]
          frame False {
            n104 = Concatenate Strings(w273, w272, w271) -> (w270:string)
          }
          frame True {
          }
        }
      }
      frame 11 {
        w294 = u32 1
        w280 = cluster{"first":u32, "second":u32} {"first"=3, "second"=2}
        # "Partial read"
        n105 = call "Create.vim"("error in (no error)"=w285, "Data Type"=w280) -> ("error out"=w287:errorcluster, "CIPC Reference"=w286:u64)  [unwired: 6 in, 2 out]
        n106 = Unbundle By Name(w280) -> ("second"=w279:u32, "first"=w277:u32)
        n107 = call "Write Element.vim"("error in (no error)"=w287, "Data in"=w280, "CIPC Reference in"=w286) -> ("error out"=w288:errorcluster, "CIPC Reference out"=w289:u64)  [unwired: 5 in, 2 out]
        n108 = call "Read Advanced.vim"("Data Element"=T1 {"Bytes to Read"=4, "Element Offset"=4}, "error in (no error)"=w288, "Data in"=w294, "CIPC Reference in"=w289) -> ("error out"=w290:errorcluster, "Data out"=w281:u32, "CIPC Reference out"=w291:u64, "Success"=w283:bool)  [unwired: 3 in, 1 out]
        n109 = Equal?(x=w281, y=w279) -> (x = y?=w275:bool)
        n110 = call "Read Advanced.vim"("Data Element"=T1 {"Bytes to Read"=4, "Element Offset"=0}, "error in (no error)"=w290, "Data in"=w294, "CIPC Reference in"=w291) -> ("error out"=w293:errorcluster, "Data out"=w278:u32, "CIPC Reference out"=w292:u64, "Success"=w282:bool)  [unwired: 3 in, 1 out]
        n111 = Equal?(x=w278, y=w277) -> (x = y?=w276:bool)
        n112 = call "Close.vi"("error in (no error)"=w293, "CIPC Reference"=w292) -> ("error out"=w284:errorcluster)  [unwired: 9 in]
        n113 = Compound Arithmetic op=AND(w283, w282, w275, w276) -> (w297:bool)
        n114 = case shown="True" w297 {
          tunnel: w301 -> [w305 w306]
          tunnel: [w302 w306] -> w300
          tunnel: "Failed partial read" -> [w304 _]
          tunnel: "\r" -> [w303 _]
          frame False {
            n115 = Concatenate Strings(w305, w304, w303) -> (w302:string)
          }
          frame True {
          }
        }
      }
      frame 12 {
        w316 = 1.0
        w309 = 0.0
        # "Read double value"
        n116 = call "Get Element Description Variant.vi"("Data Type"=w309) -> ("Encoder Data"=w308:T6)  [unwired: 8 in, 2 out]
        n117 = Unbundle By Name(w308) -> ("Data"=w307:string)
        n118 = call "Create Advanced.vim"("Encoded Data Description"=w307, "error in (no error)"=w312, "Data Type"=w309) -> ("error out"=w311:errorcluster, "CIPC Reference"=w310:u64)  [unwired: 5 in, 2 out]
        n119 = call "Write Element.vim"("error in (no error)"=w311, "Data in"=w316, "CIPC Reference in"=w310) -> ("error out"=w319:errorcluster)  [unwired: 5 in, 3 out]
        n120 = call "Read Element.vim"("error in"=w319, "Data in"=w309, "CIPC Reference in"=w310) -> ("error out"=w317:errorcluster, "Data out"=w318:dbl, "Success"=w313:bool)  [unwired: 4 in, 2 out]
        n121 = Equal?(x=w318, y=w316) -> (x = y?=w315:bool)
        n122 = call "Close.vi"("error in (no error)"=w317, "CIPC Reference"=w310) -> ("error out"=w314:errorcluster)  [unwired: 9 in]
        n123 = Compound Arithmetic op=AND(invert w314, w313, w315) -> (w320:bool)
        n124 = case shown="True" w320 {
          tunnel: w324 -> [w328 w329]
          tunnel: [w325 w329] -> w323
          tunnel: "Failed advanced create" -> [w327 _]
          tunnel: "\r" -> [w326 _]
          frame False {
            n125 = Concatenate Strings(w328, w327, w326) -> (w325:string)
          }
          frame True {
          }
        }
      }
    }
  }
  "error out" <- w1
  "status" <- w3
  n126 = And Array Elements(Boolean array=w7) -> (logical AND=→"pass":bool)
